vi "FTW-ERR-Ignore.vi"(2 "Codes to filter":i32[](array[numeric]), 5 "error to filter":errorcluster) -> (6 "filtered error":errorcluster)   [LabVIEW 2012]
panel:
  # "Inputs"
  # "Outputs"
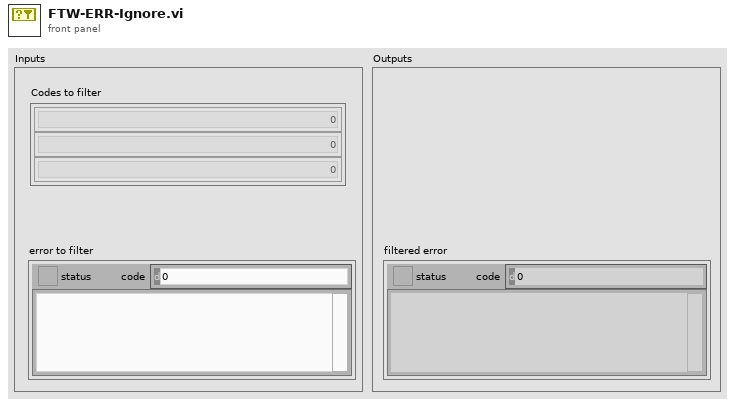
[diagram p1: front panel]
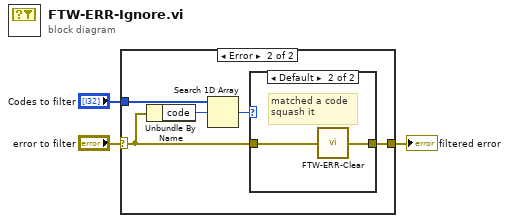
[diagram p0: block diagram]
diagram:
  n1 = case shown="Error" "error to filter" {
    selector: "error to filter" -> [w4 w8]
    tunnel: [w4 w9] -> w2
    tunnel: "Codes to filter" -> [_ w6]
    frame No Error {
    }
    frame Error {
      n2 = Unbundle By Name(w8) -> ("code"=w7:i32)
      n3 = Search 1D Array(1D array=w6, element=w7) -> (index of element=w5:i32)  [unwired: 1 in]
      n4 = case shown="Default" w5 {
        tunnel: w8 -> [w10 w12]
        tunnel: [w10 w11] -> w9
        frame -1 {
        }
        frame Default {
          # "matched a code\nsquash it"
          n5 = call "FTW-ERR-Clear.vi"("error to snuff"=w12) -> ("no error"=w11:errorcluster)
        }
      }
    }
  }
  "filtered error" <- w2
